vi "GenTables.vi"(0 "Dcs":dbl[](array[numeric])=[0.0, 0.3, 0.6], 5 "Final":dbl[](array[numeric])=[20.0, 40.0, 60.0], 7 "Start":dbl[](array[numeric])=[0.001, 0.003, 0.005], 9 "T":dbl[](array[numeric])=[50.0, 100.0, 150.0], 11 "windows":dbl[](array[numeric])=[0.0, 0.15, 0.3]) -> (4 "Array 2":T1(array[cluster]))   [LabVIEW 2014]
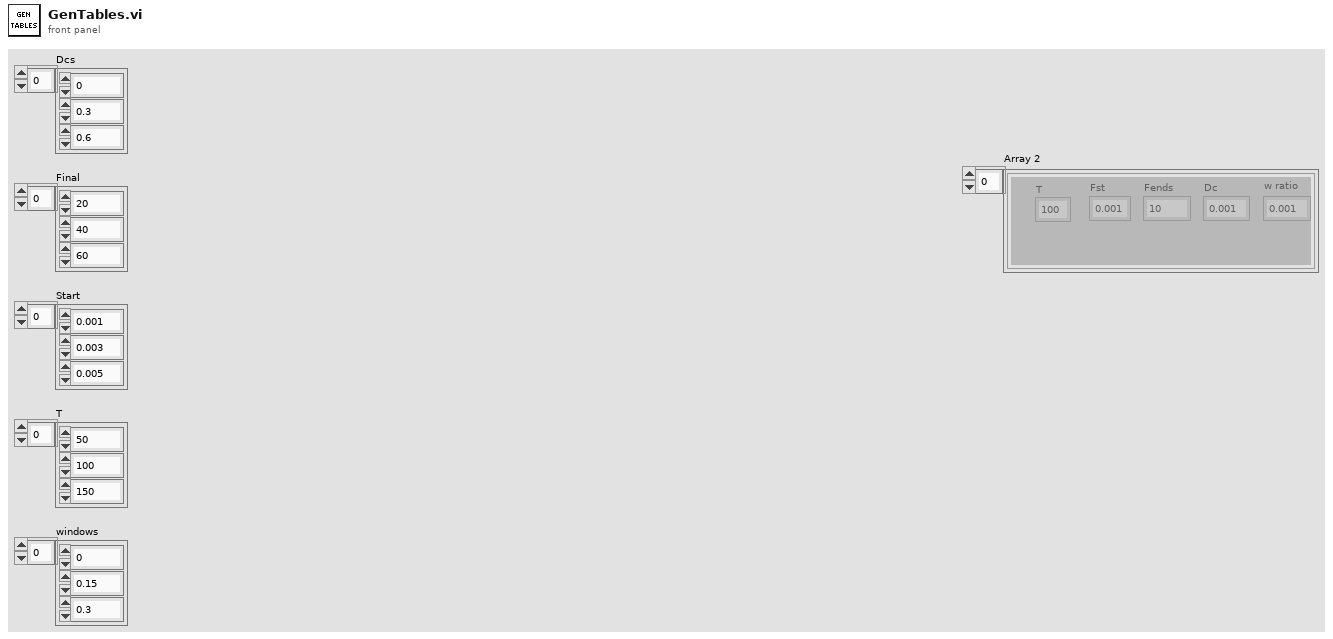
[diagram p1: front panel]
types:
  T1 = cluster{"T":dbl, "Fst":dbl, "Fends":dbl, "Dc":dbl, "w ratio":dbl}[]
  T2 = cluster{"T":dbl, "Fst":dbl, "Fends":dbl, "Dc":dbl, "w ratio":dbl}
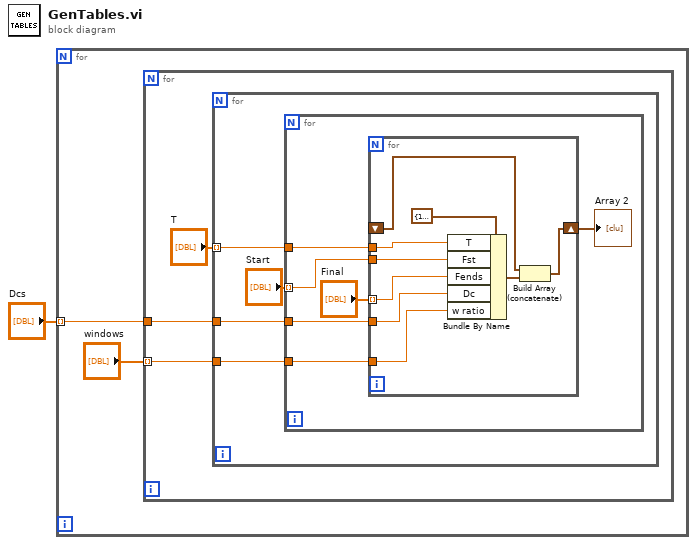
[diagram p0: block diagram]
diagram:
  n1 = for {
    tunnel: "Dcs" -> [w2] mode=indexing
    n2 = for {
      tunnel: "windows" -> [w5] mode=indexing
      tunnel: w2 -> [w4]
      n3 = for {
        tunnel: "T" -> [w9] mode=indexing
        tunnel: w5 -> [w8]
        tunnel: w4 -> [w7]
        n4 = for {
          tunnel: "Start" -> [w15] mode=indexing
          tunnel: w9 -> [w14]
          tunnel: w8 -> [w13]
          tunnel: w7 -> [w12]
          n5 = for {
            tunnel: "Final" -> [w20] mode=indexing
            tunnel: w15 -> [w19]
            tunnel: w14 -> [w18]
            shift-right: [w24] -> w11
            shift-left: _ -> [w25]
            tunnel: w13 -> [w21]
            tunnel: w12 -> [w22]
            n6 = Bundle By Name(cluster=T2 {"T"=150.0, "Fst"=0.001, "Fends"=10.0, "Dc"=0.0, "w ratio"=0.1} ("DOE parameters"), "T"=w18, "Fst"=w19, "Fends"=w20, "Dc"=w22, "w ratio"=w21) -> (w17:T2)
            n7 = Build Array (concatenate)(w25, w17) -> (w24:T1)
          }
          "Array 2" <- w11
        }
      }
    }
  }
